vi "Configure Bleeder.vi"(8 "error in (no error)":errorcluster, 10 "Enable Bleeder Circuit (T: Enable)":bool=TRUE, 11 "VISA resource name":refnum<visa-resource-name>) -> (0 "error out":errorcluster, 3 "VISA resource name out":refnum<visa-resource-name>)   [LabVIEW 2023]
doc: "Turns the bleeder on and off."
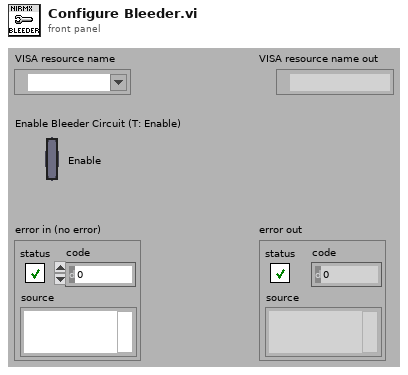
[diagram p1: front panel]
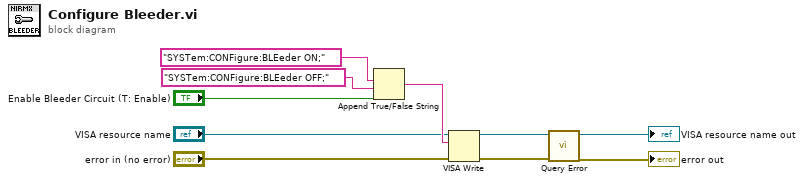
[diagram p0: block diagram]
diagram:
  n1 = Append True/False String(1:"Enable Bleeder Circuit (T: Enable)", 2:"SYSTem:CONFigure:BLEeder OFF;", 3:"SYSTem:CONFigure:BLEeder ON;") -> (0:w7:string)  [unwired: 1 in]
  n2 = VISA Write(VISA resource name="VISA resource name", write buffer=w7, error in (no error)="error in (no error)") -> (VISA resource name out=w4:refnum<visa-resource-name>, error out=w3:errorcluster)  [unwired: 1 out]
  n3 = call "Query Error.vi"("error in (no error)"=w3, "VISA resource name"=w4) -> ("error out"=→"error out":errorcluster, "VISA resource name out"=→"VISA resource name out":refnum<visa-resource-name>)  [unwired: 6 in, 2 out]
